vi "Create placeholder.vi"(11 "TEMPLATE Actor in":refnum<class "TEMPLATE Actor.lvclass">) -> (0 "Error out":errorcluster, 3 "TEMPLATE Actor out":refnum<class "TEMPLATE Actor.lvclass">)   [LabVIEW 2025, in "_Template.lvlib" / "Templates.lvlib" / "TEMPLATE Actor.lvlib" / "TEMPLATE Actor.lvclass"]
uses:
  TEMPLATE Actor.lvclass
  TEMPLATE Actor.lvclass/TEMPLATE Actor.ctl
  jettl/jettl/Actor/Actor.lvlib
  Aliases For Created.ctl
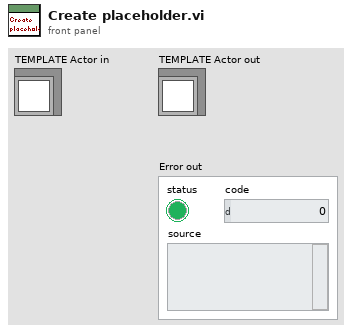
[diagram p1: front panel]
types:
  T1 = typedef "_Template.lvlib/Templates.lvlib/TEMPLATE Actor.lvlib/TEMPLATE Actor.lvclass/Aliases For Created.ctl" = enum16{""}
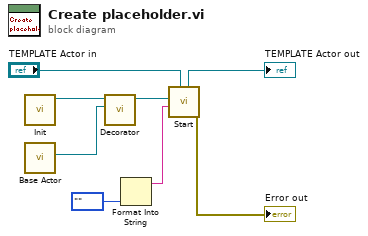
[diagram p0: block diagram]
diagram:
  n1 = call "Init.vi"() -> ("TEMPLATE Actor out"=w8:refnum<class "TEMPLATE Actor.lvclass">)  [unwired: 11 in]
  n2 = call "Base Actor.vi"() -> ("Actor"=w7:refnum<class "Actor.lvclass">)  [unwired: 11 in]
  n3 = call-dynamic "Decorator.vi"("Actor"=w7, "TEMPLATE Actor in"=w8) -> ("TEMPLATE Actor out"=w3:refnum<class "TEMPLATE Actor.lvclass">)  [unwired: 9 in]
  n4 = Format Into String(Aliases_For_Created."" ("Aliases For Created")) -> (resulting string=w2:string)  [unwired: 3 in, 1 out]
  n5 = call "Start.vi"("Actor in"="TEMPLATE Actor in", "Alias"=w2, "Actor"=w3) -> ("Error out"=→"Error out":errorcluster, "Actor out"=→"TEMPLATE Actor out":refnum<class "TEMPLATE Actor.lvclass">)  [unwired: 7 in]
